vi "DCC Set Multi Parameters.vi"(6 "DCC Data In":T1, 7 "Enable Outputs":bool, 8 "Error In":errorcluster, 10 "Module No":i16, 11 "DLL Path":path) -> (0 "Error Out":errorcluster, 2 "Module No":i16, 3 "DLL Path":path)   [LabVIEW 2019]
doc: "The procedure sends all parameters from the ‘DCCdata’ structure to the internal DLL tructures and, if ‘send_to_hard’ is equal 1, to the control registers of the DCC module ‘mod_no’.\n\nThe new parameter values are recalculated according to the parameter limits and hardware restrictions. Furthermore, cross dependencies between different parameters are taken into account to ensure the correct hardware operation. It is recommended to read back the parameters after setting to get their true values after recalculation.\nThe values of ‘base_adr’ and ‘active’ are not changed. They can be changed only by a new ini_file an a DCC_init call. If an error occurs for a particular parameter, the procedure does not set the rest of the parameters and returns with an error code. \n\nAugust 2018\nFrank Quadt & Stefan Smietana\ninfo@becker-hickl.com"
uses:
  DCC_Controls/DCC_Data_Cluster.ctl
panel:
  # "(c) 2021 Becker & Hickl GmbH\n     All Rights Reserved."
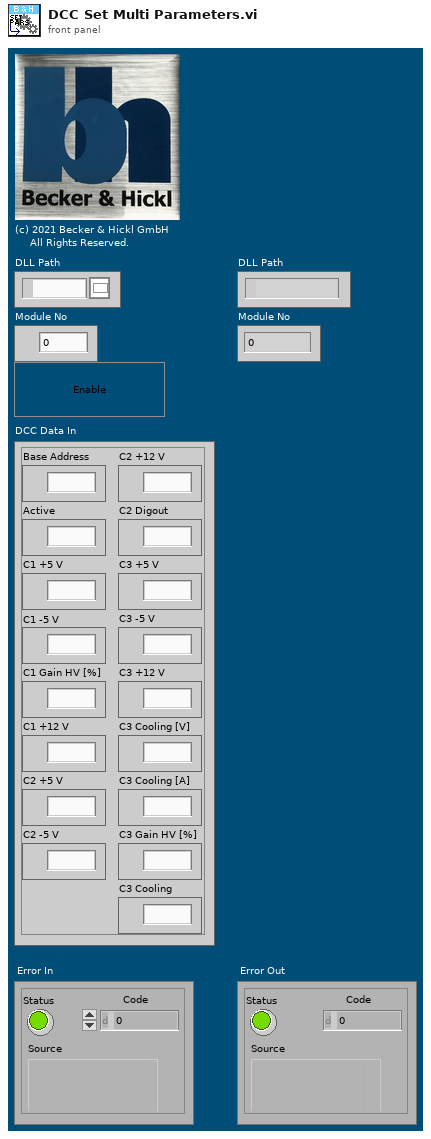
[diagram p1: front panel]
types:
  T1 = typedef "DCC_Data_Cluster.ctl" = cluster{"Base Address":u16, "Active":i16, "C1 +5 V":i16, "C1 -5 V":i16, "C1 Gain HV [%]":sgl, "C1 +12 V":i16, "C2 +5 V":i16, "C2 -5 V":i16, "C2 +12 V":i16, "C2 Digout":i16, "C3 +5 V":i16, "C3 -5 V":i16, "C3 +12 V":i16, "C3 Cooling [V]":sgl, "C3 Cooling [A]":sgl, "C3 Gain HV [%]":sgl, "C3 Cooling":i16}
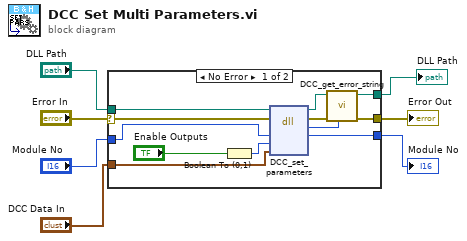
[diagram p0: block diagram]
diagram:
  n1 = case shown="No Error" "Error In" {
    selector: "Error In" -> [w19 w21]
    tunnel: [w15 w21] -> w6
    tunnel: [w14 w20] -> w5
    tunnel: "DLL Path" -> [w18 w20]
    tunnel: "DCC Data In" -> [w13 _]
    tunnel: "Module No" -> [w12 w22]
    tunnel: [w10 w22] -> w1
    frame No Error {
      n2 = Boolean To (0,1)(Boolean="Enable Outputs") -> (0, 1=w9:i16)
      n3 = dll-call lib="C:/Program Files (x86)/BH/DCC/DLL/dcc64.dll" fn="DCC_set_parameters"(path in=w18, error in=w19, "ModuleNo"=w12, "Send2Hard"=w9, "DataCluster"=w13) -> (path out=w17:path, error out=w16:errorcluster, "return type"=w11:i16, "ModuleNo"=w10:i16)  [unwired: 3 in]
      n4 = call "DCC_get_error_string.vi"("Error ID"=w11, "Error In"=w16, "DLL Path"=w17) -> ("Error Out"=w15:errorcluster, "DLL Path"=w14:path)  [unwired: 6 in, 1 out]
    }
    frame Error {
    }
  }
  "Error Out" <- w6
  "DLL Path" <- w5
  "Module No" <- w1
